vi "Create Custom Char.vi"(7 "Char #":u8, 8 "error in (no error)":errorcluster, 9 "Char":T1=[[FALSE, FALSE, FALSE, FALSE, FALSE], [FALSE, FALSE, FALSE, FALSE, FALSE], [FALSE, FALSE, FALSE, FALSE, FALSE], [FALSE, FALSE, FALSE, FALSE, FALSE], [FALSE, FALSE, FALSE, FALSE, FALSE], [FALSE, FALSE, FALSE, FALSE, FALSE], [FALSE, FALSE, FALSE, FALSE, FALSE], [FALSE, FALSE, FALSE, FALSE, FALSE]], 10 "Session In":refnum<class "Session.lvclass">, 11 "Character LCD in":refnum<class "PCF8574 I2C LCD.lvclass">) -> (0 "error out":errorcluster, 2 "Session Out":refnum<class "Session.lvclass">, 3 "Character LCD out":refnum<class "PCF8574 I2C LCD.lvclass">)   [LabVIEW 2020, in "CTI-Peripheral.lvlib" / "PCF8574 I2C LCD.lvclass"]
uses:
  PCF8574 I2C LCD.lvclass
  Character LCD/Custom Char.ctl
  CTI/Session/Session.lvclass
  HD44780 LCD/Command.ctl
  Mode.ctl
  HD44780 LCD/HD44780 LCD.lvlib
  Character LCD/Char LCD.lvclass
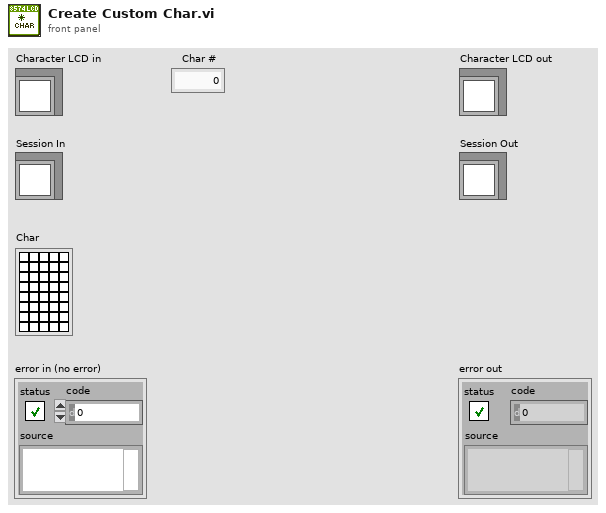
[diagram p1: front panel]
types:
  T1 = typedef "CTI-Peripheral.lvlib/Char LCD.lvclass/Custom Char.ctl" = bool[][]
  T2 = typedef "CTI-Peripheral.lvlib/HD44780 LCD.lvlib/Command.ctl" = enum16{"ClearDisplay", "ReturnHome", "EntryModeSet", "DisplayControl", "CursorShift", "FunctionSet", "SetCGRamAddr", "SetDDRamAddr"}
  T3 = typedef "CTI-Peripheral.lvlib/PCF8574 I2C LCD.lvclass/Mode.ctl" = enum8{"Command", "Character"}
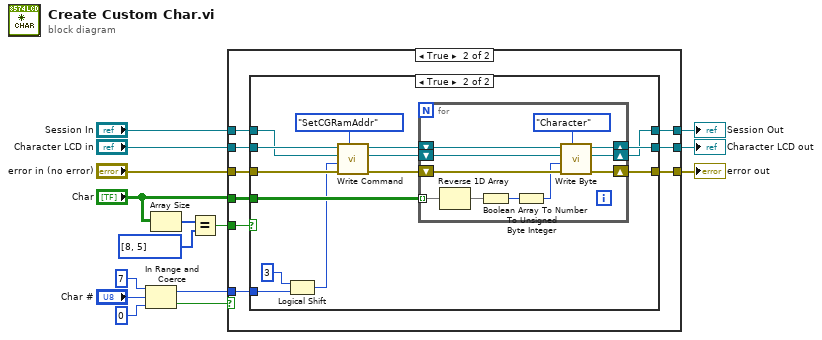
[diagram p0: block diagram]
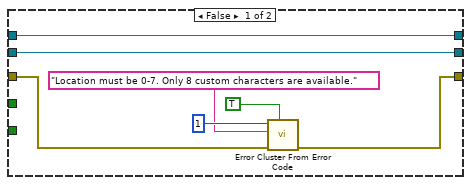
[diagram p2: hidden frame]
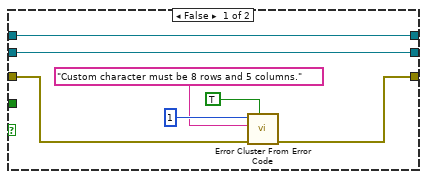
[diagram p3: hidden frame]
diagram:
  n1 = In Range and Coerce(upper limit=u8 7 ("lower limit"), x="Char #", lower limit=u8 0) -> (coerced(x)=w14:u8, In Range?=w15:bool)
  n2 = Array Size(array="Char") -> (size(s)=w13:i32[])
  n3 = Equal?(x=w13, y=i32[] [8, 5]) -> (x = y?=w9:bool)
  n4 = case shown="True" w15 {
    tunnel: w14 -> [_ w27]
    tunnel: "Character LCD in" -> [w21 w29]
    tunnel: "error in (no error)" -> [w17 w28]
    tunnel: "Char" -> [_ w31]
    tunnel: w9 -> [_ w30]
    tunnel: "Session In" -> [w22 w26]
    tunnel: [w22 w25] -> w2
    tunnel: [w21 w24] -> w4
    tunnel: [w16 w23] -> w3
    frame False {
      n5 = call <vilib>:"Error Cluster From Error Code.vi"("show call chain? (False)"=TRUE, "error in (no error)"=w17, "error message (\"\")"="Location must be 0-7. Only 8 custom characters are available.", "error code (0)"=1) -> ("error out"=w16:errorcluster)  [unwired: 5 in]
    }
    frame True {
      n6 = case shown="True" w30 {
        tunnel: w31 -> [_ w52]
        tunnel: w29 -> [w37 w49]
        tunnel: w28 -> [w33 w51]
        tunnel: w27 -> [_ w45]
        tunnel: w26 -> [w38 w46]
        tunnel: [w38 w40] -> w25
        tunnel: [w37 w43] -> w24
        tunnel: [w32 w41] -> w23
        frame False {
          n7 = call <vilib>:"Error Cluster From Error Code.vi"("show call chain? (False)"=TRUE, "error in (no error)"=w33, "error message (\"\")"="Custom character must be 8 rows and 5 columns.", "error code (0)"=1) -> ("error out"=w32:errorcluster)  [unwired: 5 in]
        }
        frame True {
          n8 = Logical Shift(y=i16 3, x=w45) -> (x << y=w42:u8)
          n9 = call "Write Command.vi"("Command"=Command."SetCGRamAddr", "error in (no error)"=w51, "Value (0)"=w42, "Session In"=w46, "PCF8574 I2C LCD in"=w49) -> ("error out"=w50:errorcluster, "Session Out"=w47:refnum<class "Session.lvclass">, "PCF8574 I2C LCD out"=w48:refnum<class "PCF8574 I2C LCD.lvclass">)  [unwired: 4 in]
          n10 = for {
            tunnel: w52 -> [w63] mode=indexing
            shift-right: [w55] -> w41
            shift-left: w50 -> [w59]
            shift-right: [w57] -> w43
            shift-left: w48 -> [w61]
            shift-right: [w56] -> w40
            shift-left: w47 -> [w60]
            n11 = Reverse 1D Array(array=w63) -> (reversed array=w54:bool[])
            n12 = Boolean Array To Number(Boolean array=w54) -> (number=w62:u32)
            n13 = To Unsigned Byte Integer(number=w62) -> (unsigned 8bit integer=w58:u8)
            n14 = call "Write Byte.vi"("Mode (Command)"=Mode."Character", "error in (no error)"=w59, "Value"=w58, "Session in"=w60, "PCF8574 I2C LCD in"=w61) -> ("error out"=w55:errorcluster, "Session out"=w56:refnum<class "Session.lvclass">, "PCF8574 I2C LCD out"=w57:refnum<class "PCF8574 I2C LCD.lvclass">)  [unwired: 4 in]
          }
        }
      }
    }
  }
  "error out" <- w3
  "Character LCD out" <- w4
  "Session Out" <- w2
